vi "Initialise Hardware Splash.vi"(8 "error in (no error)":errorcluster) -> (0 "error out":errorcluster, 2 "VISA Refnum out":refnum<visa-resource-name>, 3 "Enabled Hardware":T1={"Confocal"=TRUE, "Pinhole"=FALSE, "PIFOC"=TRUE, "Manlight"=FALSE, "iFlex"=FALSE})   [LabVIEW 2020]
panel:
  in  "animation":u16(ring)
  out "iFlex":bool
  out "Manlight":bool
  out "Pinhole":bool
  out "PIFOC":bool
  out "Confocal":bool
  out "Status":string
  in  "Start with disabled hardware":bool
  # "TweezerTron"
  # "Scanning for system hardware."
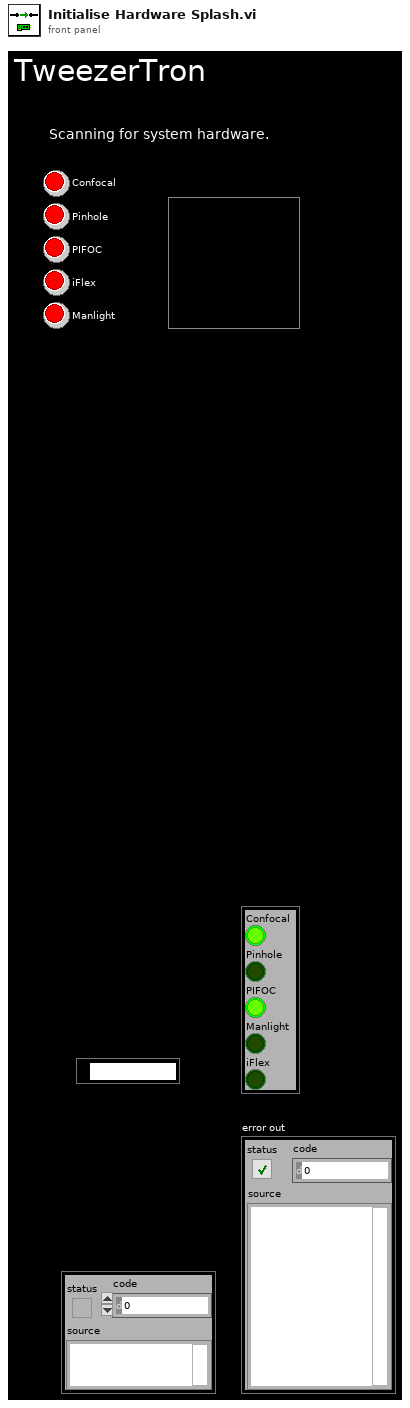
[diagram p1: front panel]
types:
  T1 = cluster{"Confocal":bool, "Pinhole":bool, "PIFOC":bool, "Manlight":bool, "iFlex":bool}
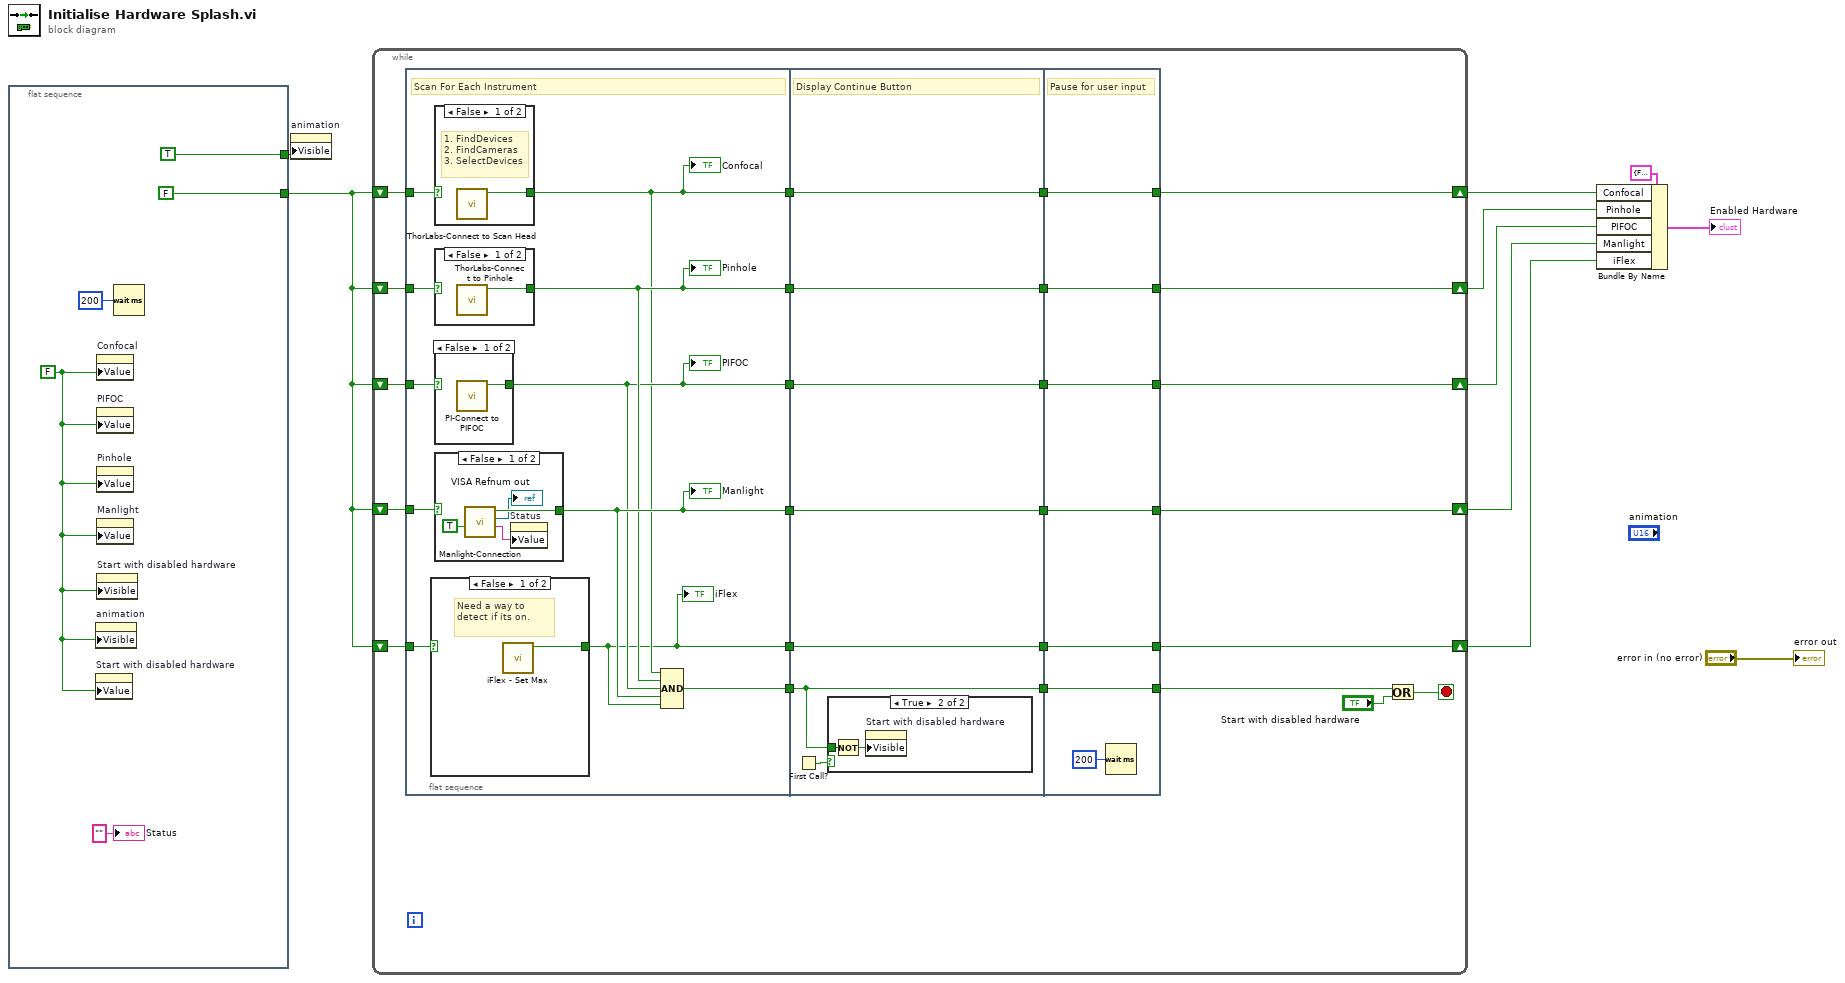
[diagram p0: block diagram]
diagram:
  n1 = flat-sequence {
    tunnel: [FALSE] -> w3
    tunnel: [TRUE ("Visible")] -> w1
    frame #0 {
      w12 = FALSE ("Confocal")
      n2 = property on="animation" class="Ring (strict)"("Visible"=w12) -> ()  [unwired: 2 in, 2 out]
      n3 = property on="Start with disabled hardware" class="Bool (strict)"("Value"=w12) -> ()  [unwired: 2 in, 2 out]
      n4 = property on="Confocal" class="Bool (strict)"("Value"=w12) -> ()  [unwired: 2 in, 2 out]
      n5 = property on="PIFOC" class="Bool (strict)"("Value"=w12) -> ()  [unwired: 2 in, 2 out]
      n6 = property on="Pinhole" class="Bool (strict)"("Value"=w12) -> ()  [unwired: 2 in, 2 out]
      n7 = property on="Manlight" class="Bool (strict)"("Value"=w12) -> ()  [unwired: 2 in, 2 out]
      n8 = property on="Start with disabled hardware" class="Bool (strict)"("Visible"=w12) -> ()  [unwired: 2 in, 2 out]
      n9 = Wait (ms)(milliseconds to wait=u32 200) -> ()  [unwired: 1 out]
      "Status" <- "" ("string")
    }
  }
  n10 = property on="animation" class="Ring (strict)"("Visible"=w1) -> ()  [unwired: 2 in, 2 out]
  n11 = while {
    shift-right: [w31] -> w9
    shift-left: w3 -> [w38]
    shift-right: [w33] -> w8
    shift-left: w3 -> [w37]
    shift-right: [w32] -> w7
    shift-left: w3 -> [w36]
    shift-right: [w34] -> w6
    shift-left: w3 -> [w35]
    shift-right: [w29] -> w2
    shift-left: w3 -> [w30]
    stop <- w40 stop-if-true
    n12 = flat-sequence {
      tunnel: w38 -> [w50]
      tunnel: w37 -> [w49]
      tunnel: w36 -> [w48]
      tunnel: w35 -> [w47]
      tunnel: w30 -> [w42]
      tunnel: [w51] -> w27
      tunnel: [w46] -> w26
      tunnel: [w45] -> w25
      tunnel: [w44] -> w24
      tunnel: [w43] -> w23
      tunnel: [w41] -> w22
      tunnel: w27 -> [w71]
      tunnel: w26 -> [w70]
      tunnel: w25 -> [w69]
      tunnel: w24 -> [w68]
      tunnel: w23 -> [w67]
      tunnel: w22 -> [w66]
      tunnel: [w71] -> w21
      tunnel: [w70] -> w20
      tunnel: [w69] -> w19
      tunnel: [w68] -> w18
      tunnel: [w67] -> w17
      tunnel: [w66] -> w16
      tunnel: [w75] -> w29
      tunnel: [w76] -> w31
      tunnel: [w77] -> w32
      tunnel: [w78] -> w33
      tunnel: [w79] -> w34
      tunnel: [w80] -> w39
      tunnel: w21 -> [w80]
      tunnel: w20 -> [w79]
      tunnel: w19 -> [w78]
      tunnel: w18 -> [w77]
      tunnel: w17 -> [w76]
      tunnel: w16 -> [w75]
      frame #0 {
        # "Scan For Each Instrument"
        n13 = case shown="False" w42 {
          selector: w42 -> [_ w53]
          tunnel: [w52 w53] -> w41
          frame False {
            # "Need a way to detect if its on."
            n14 = call "iFlex - Set Max.vi"() -> ("iFlex Enabled"=w52:bool)  [unwired: 11 in]
          }
          frame True {
          }
        }
        "iFlex" <- w41
        n15 = case shown="False" w50 {
          selector: w50 -> [_ w64]
          tunnel: [w63 w64] -> w43
          frame False {
            # "1. FindDevices\n2. FindCameras\n3. SelectDevices"
            n16 = call "ThorLabs-Connect to Scan Head.vi"() -> ("ThorLabs Scan Head Connected"=w63:bool)  [unwired: 10 in, 1 out]
          }
          frame True {
          }
        }
        "Confocal" <- w43
        n17 = case shown="False" w49 {
          selector: w49 -> [_ w62]
          tunnel: [w61 w62] -> w45
          frame False {
            n18 = call "ThorLabs-Connect to Pinhole.vi"() -> ("Thorlabs Pinhole Connected"=w61:bool)  [unwired: 10 in, 1 out]
          }
          frame True {
          }
        }
        "Pinhole" <- w45
        n19 = case shown="False" w48 {
          selector: w48 -> [_ w60]
          tunnel: [w59 w60] -> w44
          frame False {
            n20 = call "PI-Connect to PIFOC.vi"() -> ("No Errors"=w59:bool)  [unwired: 5 in, 2 out]
          }
          frame True {
          }
        }
        "PIFOC" <- w44
        n21 = case shown="False" w47 {
          selector: w47 -> [_ w58]
          tunnel: [w56 w58] -> w46
          frame False {
            n22 = call "Manlight-Connection.vi"("Connect?"=TRUE ("Connect")) -> ("Status"=w54:string, "VISA Refnum out"=→"VISA Refnum out":refnum<visa-resource-name>, "Manlight Laser Connected"=w56:bool)  [unwired: 3 in, 1 out]
            n23 = property on="Status" class="Str"("Value"=w54) -> ()  [unwired: 2 in, 2 out]
          }
          frame True {
          }
        }
        "Manlight" <- w46
        n24 = Compound Arithmetic op=AND(w43, w45, w44, w46, w41) -> (w51:bool)
      }
      frame #1 {
        # "Display Continue Button"
        n25 = First Call?() -> (First Call?: T/F=w65:bool)
        n26 = case shown="True" w65 {
          tunnel: w71 -> [_ w73]
          frame False {
          }
          frame True {
            n27 = Not(x=w73) -> (.not. x?=w72:bool)
            n28 = property on="Start with disabled hardware" class="Bool (strict)"("Visible"=w72) -> ()  [unwired: 2 in, 2 out]
          }
        }
      }
      frame #2 {
        # "Pause for user input"
        n29 = Wait (ms)(milliseconds to wait=u32 200) -> ()  [unwired: 1 out]
      }
    }
    n30 = Or(x=w39, y="Start with disabled hardware") -> (x .or. y?=w40:bool)
  }
  n31 = Bundle By Name(cluster=T1 {"Confocal"=FALSE, "Pinhole"=FALSE, "PIFOC"=FALSE, "Manlight"=FALSE, "iFlex"=FALSE} ("Enabled Hardware"), "Confocal"=w9, "Pinhole"=w8, "PIFOC"=w7, "Manlight"=w6, "iFlex"=w2) -> (→"Enabled Hardware":T1)
  "error out" <- "error in (no error)"
